vi "Widget Changes Logic.vi"(5 "Apply Pattern In":bool, 7 "Running In":bool, 8 "Execute In":cluster{"Auto":bool, "Start":bool, "Stop":bool}, 9 "Propose In":T4, 10 "Mixed Mode Widget Requests":T2={"Auto-Start Enabled"=FALSE, "Auto-Accept Enabled"=FALSE, "Exit Requested"=FALSE, "Mixed Mode Control Type"=enum."NTCP", "Input File Loaded"=FALSE, "Input File Running"=FALSE}, 11 "Mixed Mode Response Received":bool) -> (0 "Execute Out":cluster{"Auto":bool, "Start":bool, "Stop":bool}, 1 "Propose Out":T4, 2 "Mixed Mode Widget Requests Out":T2={"Auto-Start Enabled"=FALSE, "Auto-Accept Enabled"=FALSE, "Exit Requested"=FALSE, "Mixed Mode Control Type"=enum."NTCP", "Input File Loaded"=FALSE, "Input File Running"=FALSE}, 3 "Widget Changed":T1, 4 "Apply Pattern Out":bool, 6 "Running Out":bool)   [LabVIEW 2009]
uses:
  Widget Changed.ctl
  Apps/App Status Actions.ctl
  Mixed Mode Widget Button States.ctl
  Mixed Mode Control Type.ctl
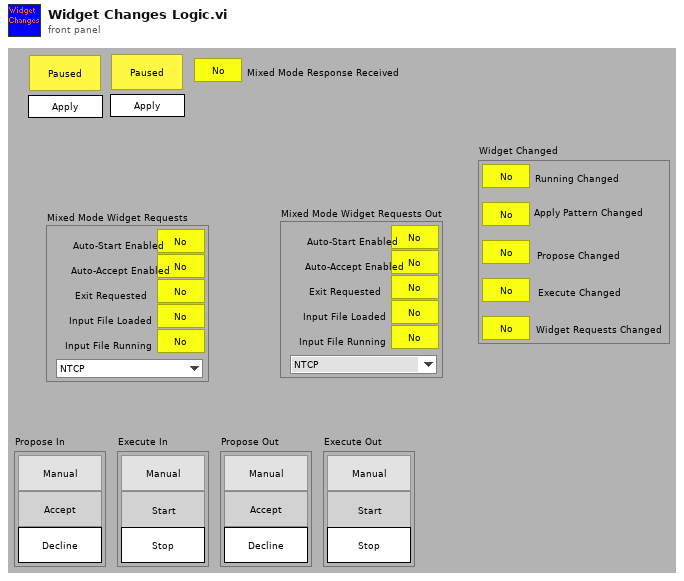
[diagram p1: front panel]
types:
  T1 = typedef "Widget Changed.ctl" = cluster{"Running Changed":bool, "Apply Pattern Changed":bool, "Propose Changed":bool, "Execute Changed":bool, "Widget Requests Changed":bool}
  T2 = typedef "Mixed Mode Widget Button States.ctl" = cluster{"Auto-Start Enabled":bool, "Auto-Accept Enabled":bool, "Exit Requested":bool, "Mixed Mode Control Type":T3, "Input File Loaded":bool, "Input File Running":bool}
  T3 = typedef "Mixed Mode Control Type.ctl" = enum32{"Manual", "Input File", "NTCP"}
  T4 = cluster{"Auto":bool, "Accept":bool, "Decline":bool}
  T5 = typedef "App Status Actions.ctl" = enum16{"Init", "Get Status", "Running", "Control", "Autobalanced", "Data Acquisition", "Set App State", "DAQ Started", "Set LBCB State", "Set All", "Set Cont Logging", "Set Step Logging", "Set MM Logging", "Set Volt Logging", "Set Cart Type", "Set DAQ Link", "Set NTCP Link"}
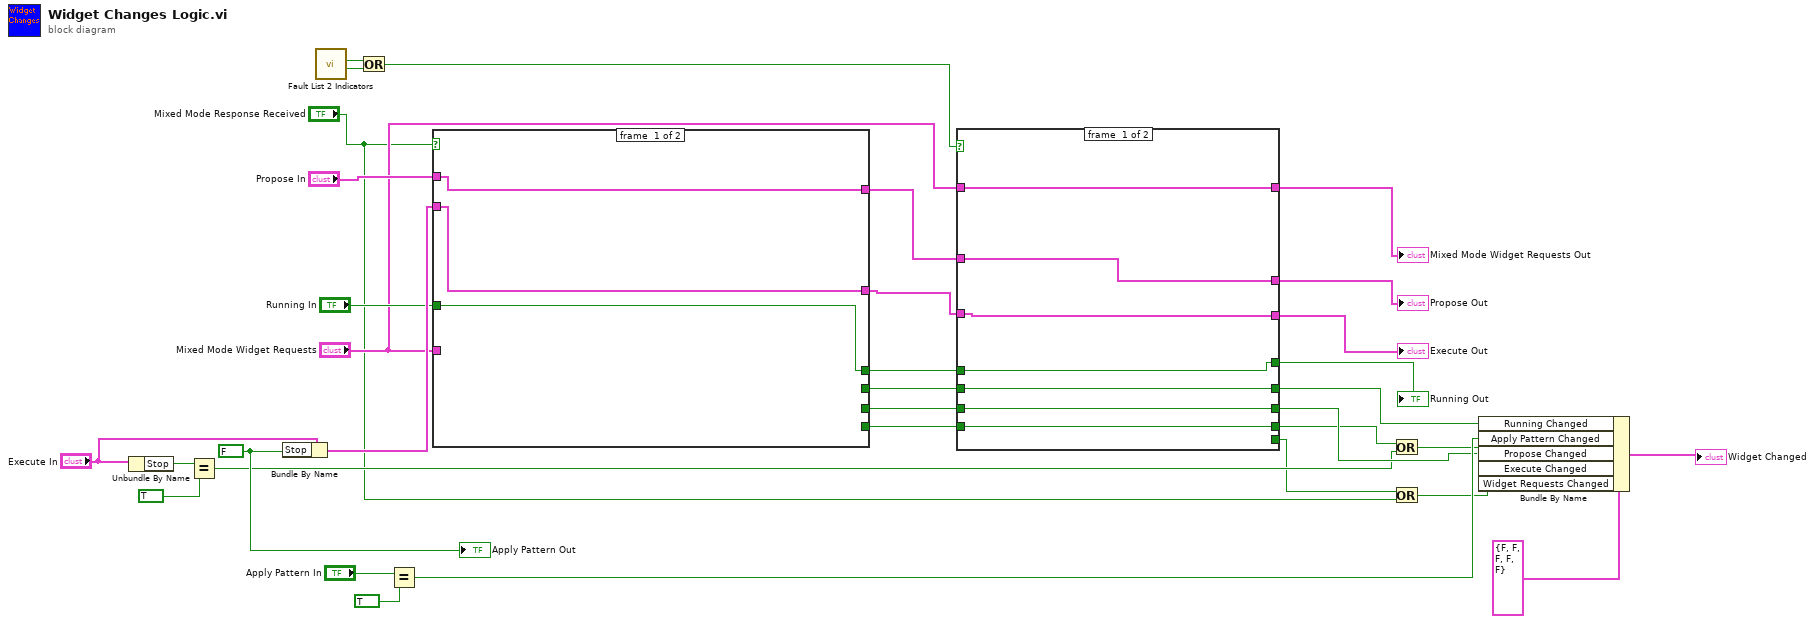
[diagram p0: block diagram]
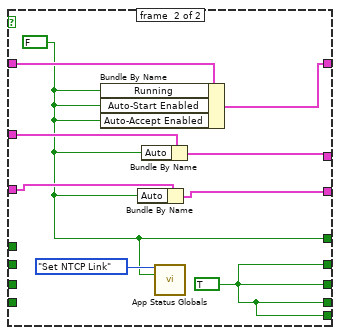
[diagram p2: hidden frame]
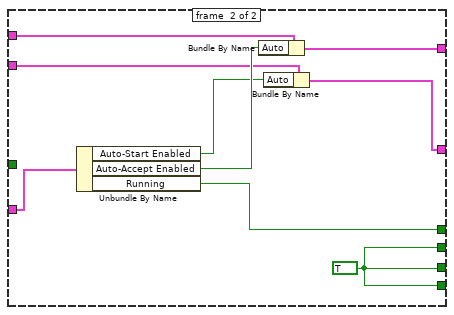
[diagram p3: hidden frame]
diagram:
  w26 = FALSE ("Stop")
  n1 = Unbundle By Name("Execute In") -> ("Stop"=w32:bool)
  n2 = Equal?(x=w32, y=TRUE) -> (x = y?=w6:bool)
  n3 = Bundle By Name(cluster="Execute In", "Stop"=w26) -> (w21:cluster{"Auto":bool, "Start":bool, "Stop":bool})
  n4 = call "Fault List 2 Indicators.vi"() -> ("Forces"=w34:bool, "Displacement"=w33:bool)  [unwired: 1 in, 9 out]
  n5 = Or(x=w33, y=w34) -> (x .or. y?=w19:bool)
  n6 = Equal?(x="Apply Pattern In", y=TRUE) -> (x = y?=w25:bool)
  n7 = case shown="False" "Mixed Mode Response Received" {
    tunnel: "Propose In" -> [w36 w45]
    tunnel: w21 -> [w37 w42]
    tunnel: "Mixed Mode Widget Requests" -> [_ w46]
    tunnel: [w36 w43] -> w18
    tunnel: [w35 w40] -> w16
    tunnel: [_ w39] -> w13
    tunnel: [_ w39] -> w14
    tunnel: [_ w39] -> w15
    tunnel: [w37 w38] -> w17
    tunnel: "Running In" -> [w35 _]
    frame #0 {
    }
    frame #1 {
      w39 = TRUE
      n8 = Unbundle By Name(w46) -> ("Auto-Start Enabled"=w41:bool, "Auto-Accept Enabled"=w44:bool, "Running"=w40:bool)
      n9 = Bundle By Name(cluster=w45, "Auto"=w44) -> (w43:T4)
      n10 = Bundle By Name(cluster=w42, "Auto"=w41) -> (w38:cluster{"Auto":bool, "Start":bool, "Stop":bool})
    }
  }
  n11 = case shown="True" w19 {
    tunnel: w18 -> [w48 w61]
    tunnel: w17 -> [w49 w62]
    tunnel: w16 -> [w50 _]
    tunnel: w15 -> [w53 _]
    tunnel: w14 -> [w52 _]
    tunnel: w13 -> [w51 _]
    tunnel: [w53 w56] -> w7
    tunnel: [w52 w56] -> w12
    tunnel: [w51 w56] -> w11
    tunnel: [w50 w54] -> w10
    tunnel: [w49 w57] -> w9
    tunnel: [w48 w58] -> w8
    tunnel: "Mixed Mode Widget Requests" -> [w47 w60]
    tunnel: [w47 w59] -> w4
    tunnel: [_ w56] -> w2
    frame #0 {
    }
    frame #1 {
      w56 = TRUE
      w54 = FALSE
      n12 = Bundle By Name(cluster=w60, "Running"=w54, "Auto-Start Enabled"=w54, "Auto-Accept Enabled"=w54) -> (w59:T2)
      n13 = Bundle By Name(cluster=w62, "Auto"=w54) -> (w57:cluster{"Auto":bool, "Start":bool, "Stop":bool})
      n14 = Bundle By Name(cluster=w61, "Auto"=w54) -> (w58:T4)
      n15 = call "App Status Globals.vi"("App Status Actions"=App_Status_Actions."Set NTCP Link", "Status\nSetting"=w54) -> ()  [unwired: 12 in, 2 out]
    }
  }
  "Execute Out" <- w9
  "Propose Out" <- w8
  "Mixed Mode Widget Requests Out" <- w4
  "Running Out" <- w10
  n16 = Or(x=w7, y=w6) -> (x .or. y?=w23:bool)
  n17 = Or(x=w2, y="Mixed Mode Response Received") -> (x .or. y?=w3:bool)
  n18 = Bundle By Name(cluster=T1 {"Running Changed"=FALSE, "Apply Pattern Changed"=FALSE, "Propose Changed"=FALSE, "Execute Changed"=FALSE, "Widget Requests Changed"=FALSE} ("Widget Changed"), "Running Changed"=w11, "Apply Pattern Changed"=w25, "Propose Changed"=w12, "Execute Changed"=w23, "Widget Requests Changed"=w3) -> (→"Widget Changed":T1)
  "Apply Pattern Out" <- w26
